vi "Father_Segmenter.vi"(3 "Threshold Percentage":dbl, 4 "FFT Size":i32, 5 "Array in":dbl[](array[numeric])) -> (0 "Merge Signals":dbl, 1 "Detected Wave":string, 2 "Dominant Frequency\nin Wave (Hz)":dbl)   [LabVIEW 2023]
panel:
  in  "Tab Control":T1(tab)
  out "Waveform Graph":cluster{i32, dbl, dbl[]}(graph)
  out "FFT Waveform Graph":dbl[](graph)
  out "Power Spectrum Graph":cluster{"f0":dbl, "df":dbl, "magnitude":dbl[]}(graph)
  out "abs(FFT) Waveform Graph":dbl[](graph)
  out "abs(FFT) Half Waveform Graph":dbl[](graph)
  out "Frequency Bins(start)":i32
  out "Frequency Bins(end)":i32
  out "Starting Frequency\nin Wave (Hz)":dbl
  out "Ending Frequency\nin Wave (Hz)":dbl
  out "Dominant Bin Location":i32
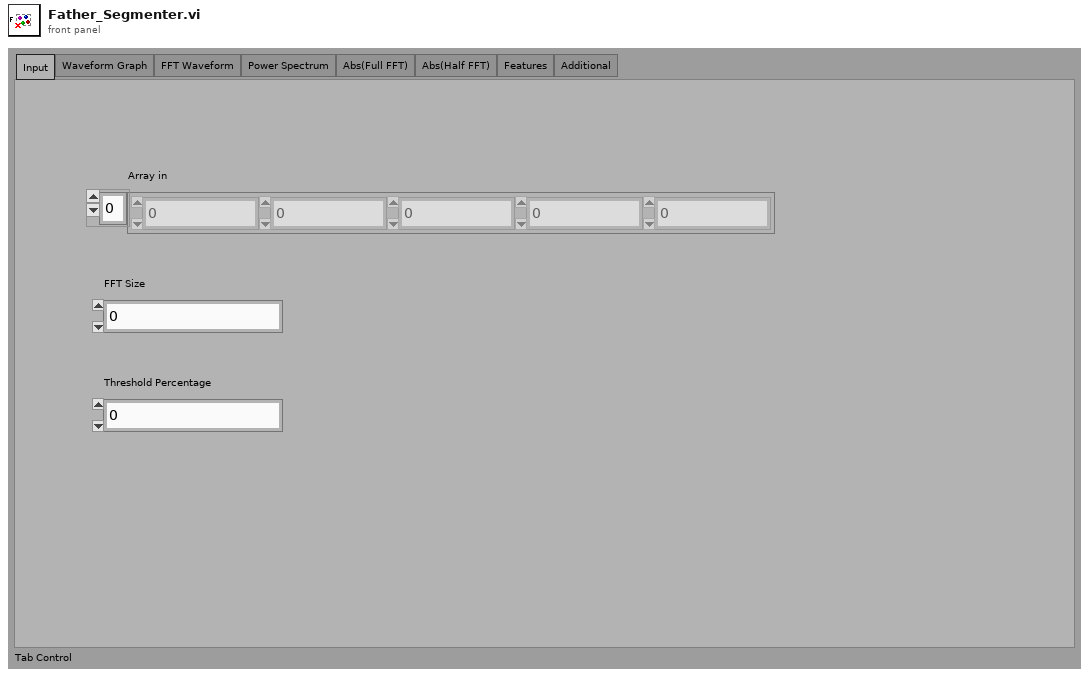
[diagram p1: front panel]
types:
  T1 = enum32{"Input", "Waveform Graph", "FFT Waveform", "Power Spectrum", "Abs(Full FFT)", "Abs(Half FFT)", "Features", "Additional"}
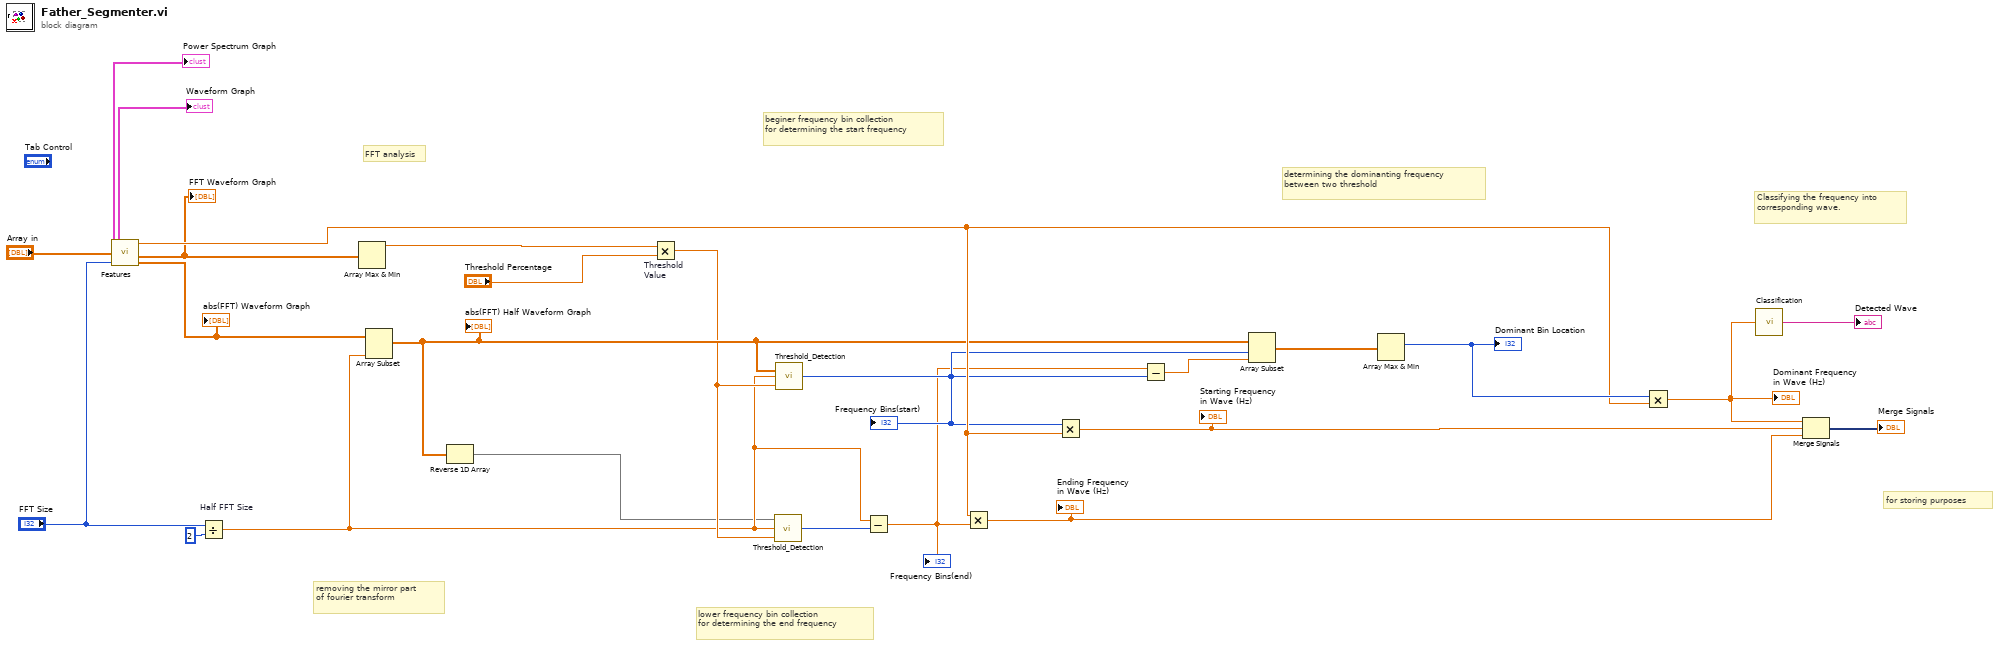
[diagram p0: block diagram]
diagram:
  # "FFT analysis"
  # "Classifying the frequency into\ncorresponding wave."
  # "for storing purposes"
  # "determining the dominanting frequency\nbetween two threshold"
  # "beginer frequency bin collection\nfor determining the start frequency"
  # "lower frequency bin collection\nfor determining the end frequency"
  # "removing the mirror part\nof fourier transform"
  n1 = call "Features.vi"("Array in"="Array in", "Sampling"="FFT Size") -> ("Power Spectrum Graph"=→"Power Spectrum Graph":cluster{"f0":dbl, "df":dbl, "magnitude":dbl[]}, "Waveform Graph"=→"Waveform Graph":cluster{i32, dbl, dbl[]}, "Frequency Resolution"=w23:dbl, "FFT"=w3:dbl[], "abs(FFT)"=w8:dbl[])  [unwired: 2 in, 1 out]
  "FFT Waveform Graph" <- w3
  "abs(FFT) Waveform Graph" <- w8
  n2 = Divide "Half FFT Size"(x="FFT Size", y=2) -> (x/y=w15:dbl)
  n3 = Array Max & Min(array=w3) -> (max value=w12:dbl)  [unwired: 3 out]
  n4 = Array Subset "Array Subset"(array=w8, length=w15) -> (w18:dbl[])  [unwired: 1 in]
  "abs(FFT) Half Waveform Graph" <- w18
  n5 = Reverse 1D Array(array=w18) -> (reversed array=w13:dbl[])
  n6 = Multiply "Threshold\nValue"(x=w12, y="Threshold Percentage") -> (x*y=w16:dbl)
  n7 = call "Threshold_Detection.vi"("Threshold Value"=w16, "Length of Array"=w15, "Array"=w13) -> ("Detection Index"=w14:i32)
  n8 = call "Threshold_Detection.vi"("Threshold Value"=w16, "Length of Array"=w15, "Array"=w18) -> ("Detection Index"=w21:i32)
  "Frequency Bins(start)" <- w21
  n9 = Subtract(x=w15, y=w14) -> (x-y=w20:dbl)
  "Frequency Bins(end)" <- w20
  n10 = Multiply(x=w23, y=w20) -> (x*y=w5:dbl)
  "Ending Frequency\nin Wave (Hz)" <- w5
  n11 = Multiply(x=w21, y=w23) -> (x*y=w6:dbl)
  "Starting Frequency\nin Wave (Hz)" <- w6
  n12 = Subtract(x=w20, y=w21) -> (x-y=w19:dbl)
  n13 = Array Subset "Array Subset"(array=w18, index=w21, length=w19) -> (w22:dbl[])
  n14 = Array Max & Min(array=w22) -> (max index (indices)=w24:i32)  [unwired: 3 out]
  "Dominant Bin Location" <- w24
  n15 = Multiply(x=w24, y=w23) -> (x*y=w7:dbl)
  "Dominant Frequency\nin Wave (Hz)" <- w7
  n16 = call "Classification.vi"("Numeric"=w7) -> ("Detected Wave"=→"Detected Wave":string)
  n17 = Merge Signals(w7, w6, w5) -> (→"Merge Signals":dynamicdata)
